vi "CreatGlobalCollector.vi"(0 "reference in":refnum<class "DAQ_Base.lvclass">, 5 "error in (no error)":errorcluster) -> (14 "reference out":refnum<class "DAQ_Base.lvclass">, 19 "error out":errorcluster)   [LabVIEW 2020, in "DAQ_Base.lvclass"]
uses:
  DAQ_Base.lvclass
  subvi/GlobalData_operation.ctl
panel:
  in  "ChannelNbr":i32=10
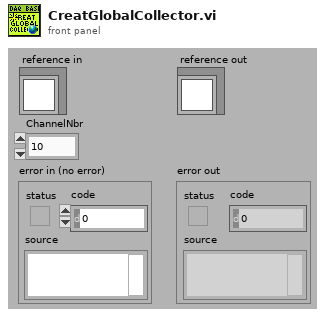
[diagram p1: front panel]
types:
  T1 = typedef "GlobalData_operation.ctl" = enum16{"idle", "read", "write", "clear", "init", "destroy"}
  T2 = typedef "DAQ_Base.lvclass/ObjectAttributesRef.ctl" = refnum<data-value>
  T3 = typedef "DAQ_Base.lvclass/ObjectAttributes.ctl" = cluster{"MyAttribute":dbl, "RootPath":path, "DAQSettings":T4, "DaqCollector":cluster{"CollectDataQueue":refnum<queue>, "ArryDataCollectorChannel":T10[], "RealTimeValues":dbl[]}, "CollectorChannelEnable":bool[]}
  T4 = typedef "DAQ_Base.lvclass/DAQSettings.ctl" = cluster{"SampleSettings":T5, "AI_ChannelSettings":T6, "AO_ChannelSettings":T8, "Cnt_ChannelSettings":T9}
  T5 = typedef "DAQ_Base.lvclass/SampleSettings.ctl" = cluster{"samples per channel":i32, "SampleRate":dbl, "TansMaxLength":dbl, "ReadTimeOut":dbl, "时钟源":tag}
  T6 = typedef "DAQ_Base.lvclass/AI_ChannelSettings.ctl" = cluster{"AI_SettingsArry":cluster{"DeviceName":tag, "physical channels":tag, "AssignName":string, "输入信号类型":T7, "Max_value":dbl, "Min_value":dbl, "单位":i32, "shunt resistor location":i32, "external shunt resistor value":dbl, "标定系数":cluster{"Scale":dbl, "Offset":dbl}}[]}
  T7 = typedef "AI信号类型.ctl" = i32
  T8 = typedef "DAQ_Base.lvclass/AO_ChannelSettings.ctl" = cluster{"布尔":bool}
  T9 = typedef "DAQ_Base.lvclass/Cnt_ChannelSettings.ctl" = cluster{"Cnt_ChannelSettings":cluster{"类型":enum16{"Linear", "Rotate"}, "CounterNbr":tag, "AssignName":string, "单位":u16, "decoding type":u16, "PPR_DistancePerPulse":dbl, "Initial Position ":dbl, "z index enable":bool, "z index phase":i32, "source":tag}[]}
  T10 = typedef "DAQ_Base.lvclass/DataCollector.ctl" = cluster{"DataCollectArry":dbl[][], "Update":bool}
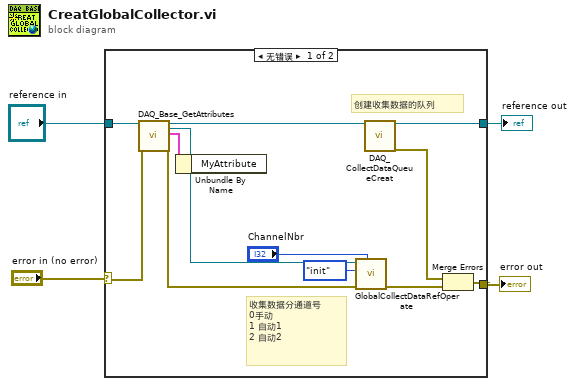
[diagram p0: block diagram]
diagram:
  n1 = case shown="无错误" "error in (no error)" {
    selector: "error in (no error)" -> [w14 w18]
    tunnel: [w16 w18] -> w3
    tunnel: [w6 w17] -> w1
    tunnel: "reference in" -> [w15 w17]
    frame No Error {
      # "收集数据分通道号\n0手动\n1 自动1\n2 自动2"
      # "创建收集数据的队列"
      n2 = call "DAQ_Base_GetAttributes.vi"("reference in"=w15, "error in (no error)"=w14) -> ("reference out"=w7:refnum<class "DAQ_Base.lvclass">, "attributes ref"=w12:T2, "attributes"=w13:T3, "error out"=w9:errorcluster)  [unwired: 14 in]
      n3 = Unbundle By Name(w13) -> ()  [unwired: 1 out]
      n4 = call "GlobalCollectDataRefOperate.vi"("ChannelNbr"="ChannelNbr", "error in (no error)"=w9, "operation"=GlobalData_operation."init", "attributes ref"=w12) -> ("error out"=w8:errorcluster)  [unwired: 5 in, 2 out]
      n5 = call-dynamic "DAQ_CollectDataQueueCreat.vi"("reference in"=w7) -> ("reference out"=w6:refnum<class "DAQ_Base.lvclass">, "error out"=w5:errorcluster)  [unwired: 17 in]
      n6 = Merge Errors(w5, w8) -> (w16:errorcluster)
    }
    frame Error {
    }
  }
  "error out" <- w3
  "reference out" <- w1
